vi "Validate_VI_Can_Be_Inlined_In_Build.vi"(5 "topLevel":bool, 6 "VI refnum in":refnum<vi>, 7 "sourceInclusion":T1, 8 "error in (no error)":errorcluster, 10 "saveLevel":u32, 11 "Build in":refnum<class "AB_PackedLibrary.lvclass">) -> (0 "error out":errorcluster, 3 "Build out":refnum<class "AB_PackedLibrary.lvclass">)   [LabVIEW 2020, in "AB_PackedLibrary.lvclass"]
uses:
  <vilib>/AppBuilder/AB_Classes/PackedLib/AB_PackedLibrary.lvclass
  <vilib>/AppBuilder/AB_Source_Inclusion.ctl
  <vilib>/AppBuilder/AB_Classes/PackedLib/AB_PackedLibrary.lvclass/AB_PackedLibrary.ctl
  <resource>/Framework/Providers/Common/provcom_StringGlobals.vi
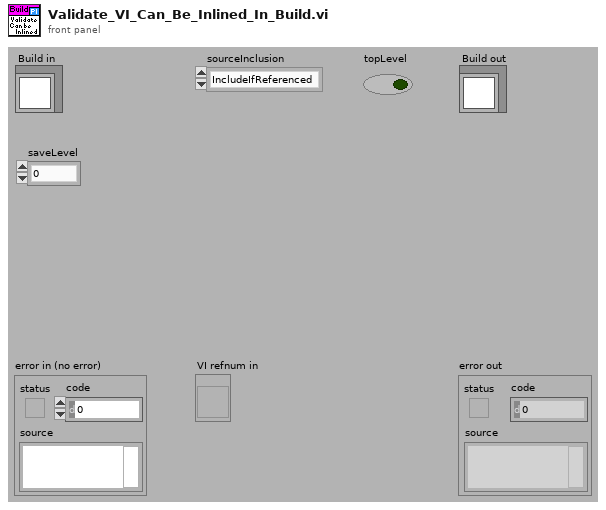
[diagram p1: front panel]
types:
  T1 = typedef "AB_Source_Inclusion.ctl" = enum16{"IncludeIfReferenced", "Include", "Exclude", "TopLevel"}
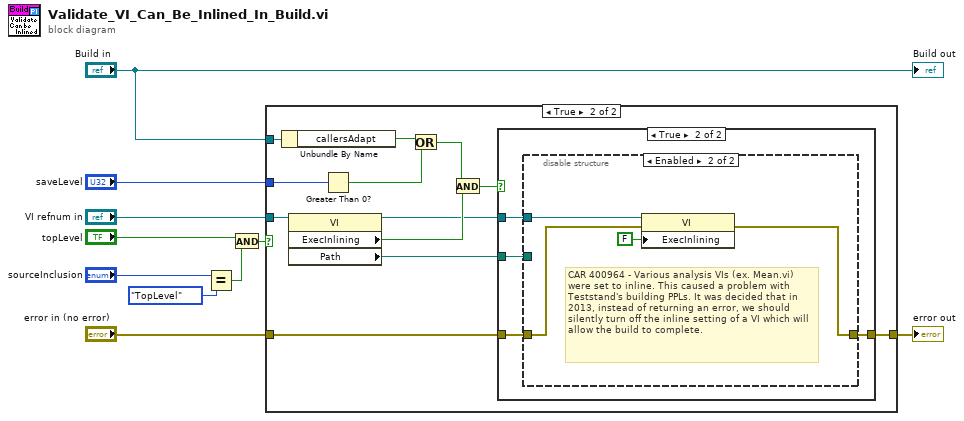
[diagram p0: block diagram]
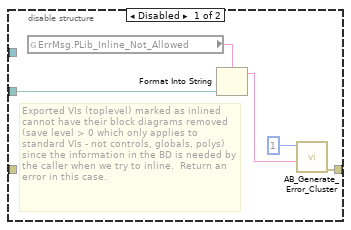
[diagram p4: hidden frame]
diagram:
  n1 = Equal?(x="sourceInclusion", y=AB_Source_Inclusion."TopLevel") -> (x = y?=w2:bool)
  n2 = And(x="topLevel", y=w2) -> (x .and. y?=w4:bool)
  n3 = case shown="True" w4 {
    tunnel: "saveLevel" -> [_ w23]
    tunnel: "error in (no error)" -> [w11 w22]
    tunnel: [w11 w21] -> w8
    tunnel: "VI refnum in" -> [_ w15]
    tunnel: "Build in" -> [_ w19]
    frame False {
    }
    frame True {
      n4 = Unbundle By Name(w19) -> ("callersAdapt"=w18:bool)
      n5 = property class="VI"(reference=w15) -> (reference out=w12:refnum<vi>, "ExecInlining"=w13:bool, "Path"=w14:path)  [unwired: 1 in, 1 out]
      n6 = Greater Than 0?(x=w23) -> (x > 0?=w17:bool)
      n7 = Or(x=w18, y=w17) -> (x .or. y?=w16:bool)
      n8 = And(x=w16, y=w13) -> (x .and. y?=w20:bool)
      n9 = case shown="True" w20 {
        tunnel: w22 -> [w24 w25]
        tunnel: [w24 w28] -> w21
        tunnel: w14 -> [_ w27]
        tunnel: w12 -> [_ w26]
        frame False {
        }
        frame True {
          n10 = disable-structure shown="Enabled" {
            disable-tunnel: [w32 w34] -> w28
            disable-tunnel: w27 -> [w30 _]
            disable-tunnel: w26 -> [_ w37]
            disable-tunnel: w25 -> [_ w35]
            frame Disabled {
              # "Exported VIs (toplevel) marked as inlined cannot have their block diagrams removed (save level > 0 which only applies to standard VIs - not controls, globals, polys) since the information in the BD is needed by the caller when we try to inline.  Return an error in this case."
              n11 = global read "provcom_StringGlobals.vi" "ErrMsg.PLib_Inline_Not_Allowed"() -> (w31:string)
              n12 = Format Into String(format string=w31, w30) -> (resulting string=w29:string)  [unwired: 2 in, 1 out]
              n13 = call <vilib>:"AB_Generate_Error_Cluster.vi"("Additional Message"=w29, "Code"=1) -> ("error out"=w32:errorcluster)  [unwired: 2 in, 7 out]
            }
            frame Enabled {
              # "CAR 400964 - Various analysis VIs (ex. Mean.vi) were set to inline. This caused a problem with Teststand's building PPLs. It was decided that in 2013, instead of returning an error, we should silently turn off the inline setting of a VI which will allow the build to complete."
              n14 = property class="VI"(reference=w37, error in=w35, "ExecInlining"=FALSE ("Execution:Inline SubVI")) -> (error out=w34:errorcluster)  [unwired: 1 out]
            }
          }
        }
      }
    }
  }
  "error out" <- w8
  "Build out" <- "Build in"
